vi "LittleBoatHindbrainSense.vi"(8 "Image Path":T1, 9 "Hindbrain Queue Cluster":T5, 10 "XBee Serial Port":refnum<visa-resource-name>, 11 "Session In":T2) -> (0 "error out":errorcluster)   [LabVIEW 2013]
uses:
  Data/TypeDefs/GPS-Compass Queue Cluster.ctl
  Data/TypeDefs/UTM Location.ctl
  Data/TypeDefs/WindData Queue Cluster.ctl
  <vilib>/vision/Image Controls.llb/IMAQ Image.ctl
  <vilib>/userdefined/High Color/IMAQdx.ctl
  <vilib>/vision/driver/NI_Vision_Acquisition_Software.lvlib
  <vilib>/vision/NI_Vision_Development_Module.lvlib
panel:
  out "Image":T1(plugin-control)
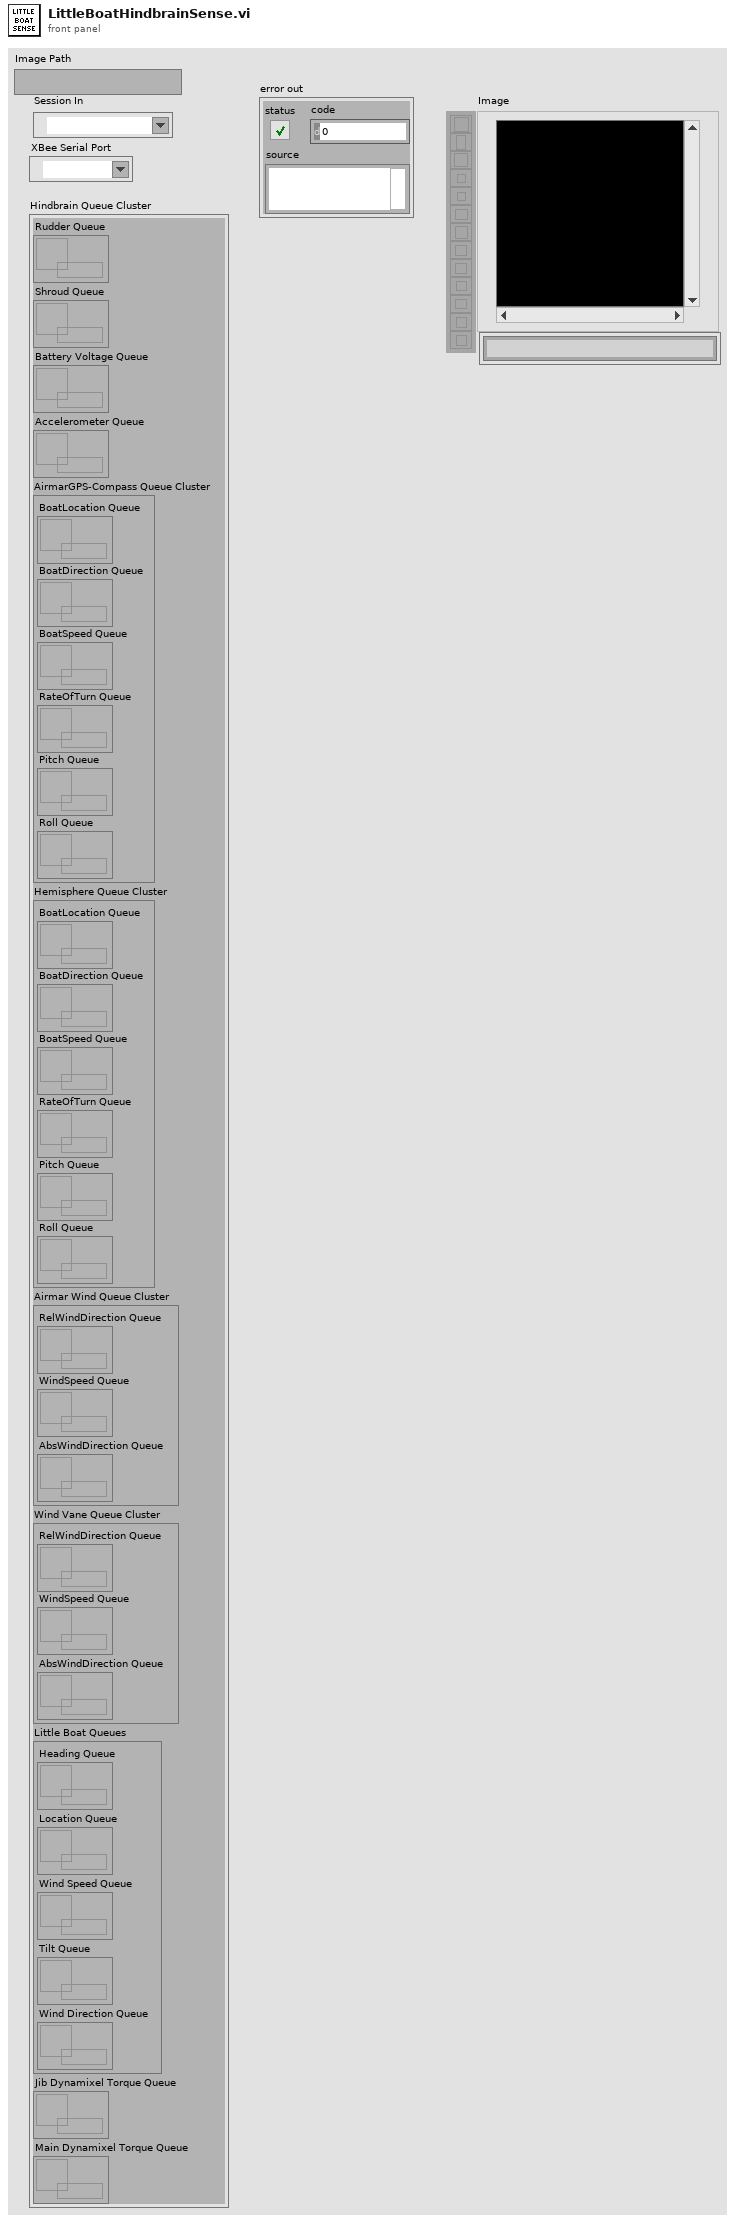
[diagram p1: front panel]
types:
  T1 = typedef "IMAQ Image.ctl" = refnum<image>
  T2 = typedef "IMAQdx.ctl" = refnum<k21>
  T3 = typedef "GPS-Compass Queue Cluster.ctl" = cluster{"BoatLocation Queue":refnum<queue>, "BoatDirection Queue":refnum<queue>, "BoatSpeed Queue":refnum<queue>, "RateOfTurn Queue":refnum<queue>, "Pitch Queue":refnum<queue>, "Roll Queue":refnum<queue>}
  T4 = typedef "WindData Queue Cluster.ctl" = cluster{"RelWindDirection Queue":refnum<queue>, "WindSpeed Queue":refnum<queue>, "AbsWindDirection Queue":refnum<queue>}
  T5 = cluster{"Rudder Queue":refnum<queue>, "Shroud Queue":refnum<queue>, "Battery Voltage Queue":refnum<queue>, "Accelerometer Queue":refnum<queue>, "AirmarGPS-Compass Queue Cluster":T3, "Hemisphere Queue Cluster":T3, "Airmar Wind Queue Cluster":T4, "Wind Vane Queue Cluster":T4, "Little Boat Queues":cluster{"Heading Queue":refnum<queue>, "Location Queue":refnum<queue>, "Wind Speed Queue":refnum<queue>, "Tilt Queue":refnum<queue>, "Wind Direction Queue":refnum<queue>}, "Jib Dynamixel Torque Queue":refnum<queue>, "Main Dynamixel Torque Queue":refnum<queue>}
  T6 = typedef "UTM Location.ctl" = cluster{"UTM Zone":dbl, "Hemisphere":enum16{"North", "South"}, "East":dbl, "North":dbl}
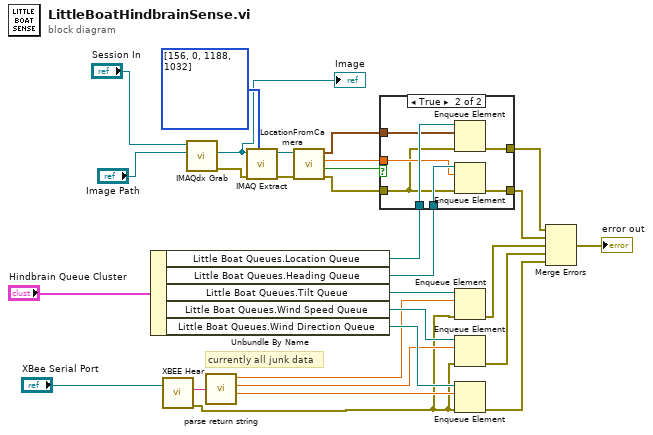
[diagram p0: block diagram]
diagram:
  # "currently all junk data"
  n1 = Unbundle By Name("Hindbrain Queue Cluster") -> ("Little Boat Queues.Location Queue"=w17:refnum<queue>, "Little Boat Queues.Heading Queue"=w16:refnum<queue>, "Little Boat Queues.Tilt Queue"=w18:refnum<queue>, "Little Boat Queues.Wind Speed Queue"=w20:refnum<queue>, "Little Boat Queues.Wind Direction Queue"=w22:refnum<queue>)
  n2 = call "XBEE Hear.vi"("VISA resource name"="XBee Serial Port") -> ("String Received"=w14:string, "error out"=w2:errorcluster)  [unwired: 1 in, 2 out]
  n3 = call <vilib>:"IMAQdx Grab.vi"("Image In"="Image Path", "Session In"="Session In") -> ("error out"=w3:errorcluster, "Image Out"=w1:T1)  [unwired: 6 in, 2 out]
  "Image" <- w1
  n4 = call "parse return string.vi"("Return String"=w14) -> ("Tilt"=w19:dbl, "Wind Speed"=w21:dbl, "Wind Direction"=w23:dbl)  [unwired: 1 out]
  n5 = call "IMAQ Extract"("Optional Rectangle"=i32[] [156, 0, 1188, 1032], "error in (no error)"=w3, "Image Src"=w1) -> ("error out"=w4:errorcluster, "Image Dst Out"=w6:T1)  [unwired: 7 in]
  n6 = call "LocationFromCamera.vi"("error in"=w4, "Image Path"=w6) -> ("error out"=w11:errorcluster, "Valid?"=w12:bool, "Angle"=w9:sgl, "Location"=w10:T6)  [unwired: 6 in]
  n7 = case shown="True" w12 {
    tunnel: [w30 w37] -> w26
    tunnel: [w30 w36] -> w25
    tunnel: w17 -> [_ w35]
    tunnel: w16 -> [_ w34]
    tunnel: w11 -> [w30 w31]
    tunnel: w10 -> [_ w33]
    tunnel: w9 -> [_ w32]
    frame False {
    }
    frame True {
      n8 = Enqueue Element(queue=w35, element=w33, error in (no error)=w31) -> (error out=w36:errorcluster)  [unwired: 1 in, 2 out]
      n9 = Enqueue Element(queue=w34, element=w32, error in (no error)=w31) -> (error out=w37:errorcluster)  [unwired: 1 in, 2 out]
    }
  }
  n10 = Enqueue Element(queue=w18, element=w19, error in (no error)=w2) -> (error out=w27:errorcluster)  [unwired: 1 in, 2 out]
  n11 = Enqueue Element(queue=w20, element=w21, error in (no error)=w2) -> (error out=w28:errorcluster)  [unwired: 1 in, 2 out]
  n12 = Enqueue Element(queue=w22, element=w23, error in (no error)=w2) -> (error out=w29:errorcluster)  [unwired: 1 in, 2 out]
  n13 = Merge Errors(w25, w26, w27, w28, w29) -> (→"error out":errorcluster)
